vi "Analog_Hysteresis.vi"() -> ()   [LabVIEW 2011]
uses:
  <vilib>/Platform/TimedLoop/XDataNode/timing_clust.ctl
  <vilib>/Platform/TimedLoop/XDataNode/nitl_modes.ctl
  <vilib>/Platform/TimedLoop/XDataNode/wakeup.ctl
  <vilib>/Utility/error.llb/DialogType.ctl
  <vilib>/DAQmx/read.llb/DAQmx Read (Analog 2D DBL NChan NSamp).vi
  <vilib>/DAQmx/write.llb/DAQmx Write (Analog 1D DBL NChan 1Samp).vi
  <vilib>/DAQmx/create/channels.llb/DAQmx Create Channel (AI-Voltage-Basic).vi
  <vilib>/DAQmx/configure/timing.llb/DAQmx Timing (Sample Clock).vi
  <vilib>/Utility/file.llb/Write To Spreadsheet File (DBL).vi
  <vilib>/DAQmx/miscellaneous.llb/DAQmx Fill In Error Info.vi
  <vilib>/Platform/TimedLoop/XDataNode/XDataNode.xnode
  <vilib>/Platform/TimedLoop/XDataNode/XDNodeRunTimeDep.lvlib
panel:
  in  "Increase":bool
  in  "Decrease":bool
  out "Displacement input":T1(graph)
  out "XY Graph":cluster{"Y":dbl[], "Y":dbl[]}[](graph)
  in  "En H Inv":bool
  out "Time":dbl
  in  "Frequency 3":dbl=1.0
  in  "Amplitude":dbl[](array[numeric])=[0.0, 0.0, 0.0]
  out "Piezo driver input":T1(graph)
  out "Capacitive Sensor":T2(graph)
  in  "stop":bool
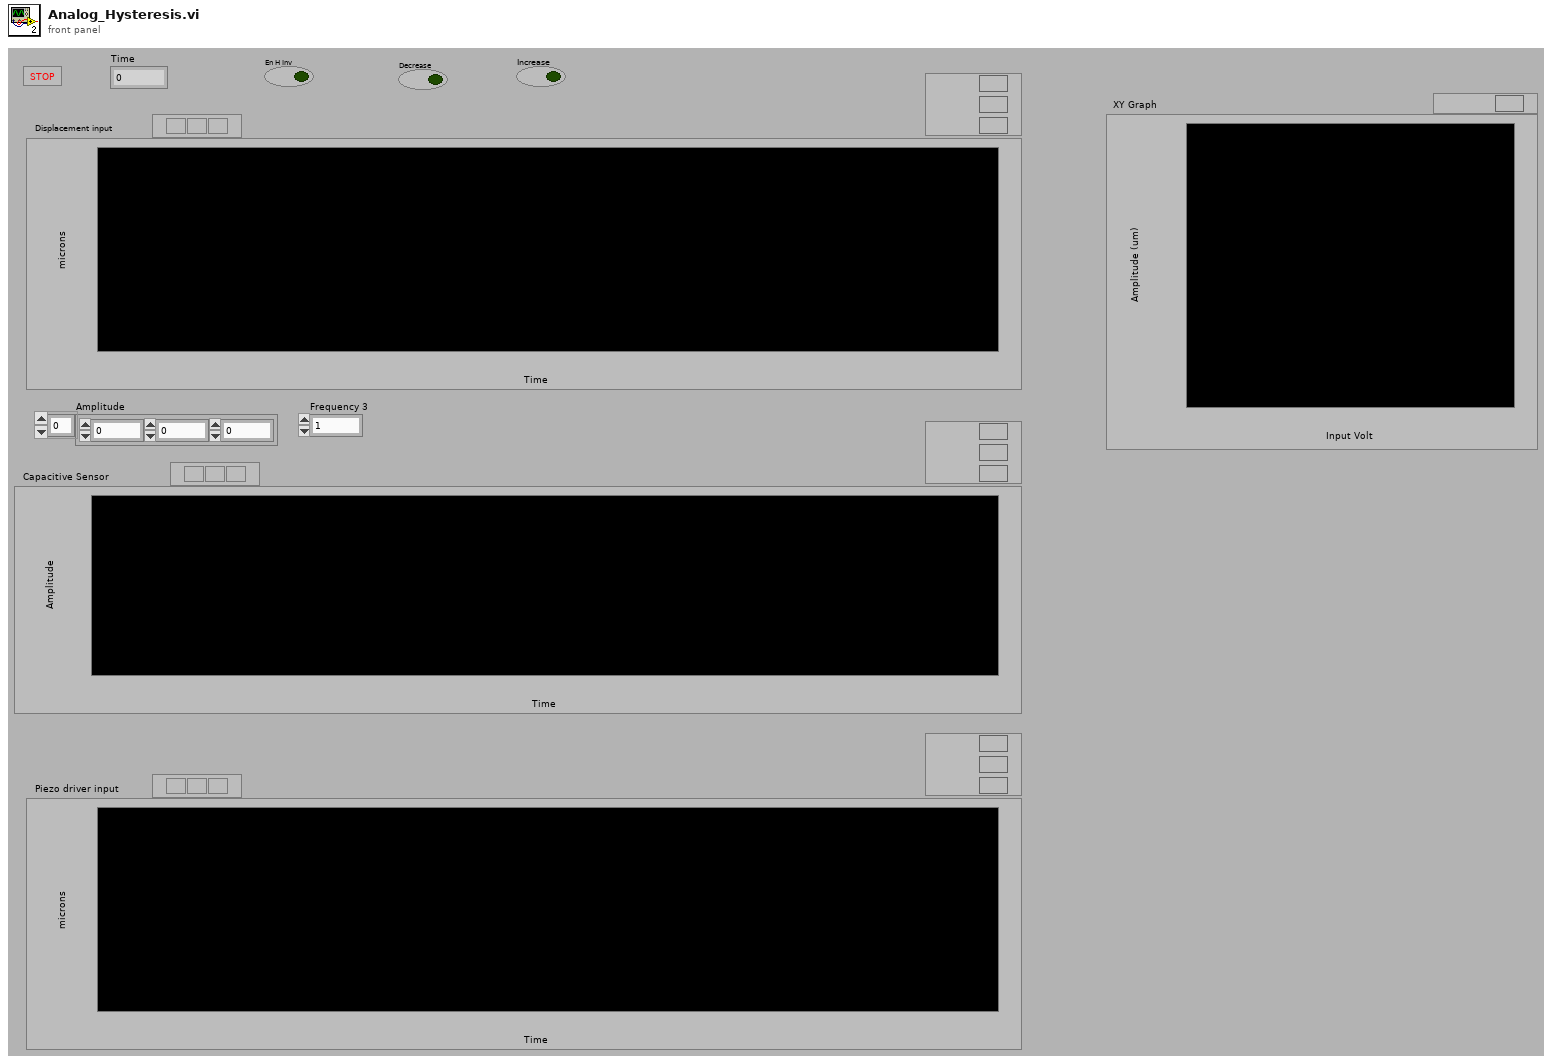
[diagram p1: front panel]
types:
  T1 = cluster{"dataOut[0]":dbl, "dataOut[1]":dbl, "dataOut[2]":dbl, "dataOut[3]":dbl, "dataOut[4]":dbl, "dataOut[5]":dbl, "dataOut[6]":dbl, "dataOut[7]":dbl, "dataOut[8]":dbl}
  T2 = cluster{"[0]":dbl, "[1]":dbl, "[2]":dbl, "[3]":dbl, "[4]":dbl, "[5]":dbl, "[6]":dbl, "[7]":dbl, "[8]":dbl}
  T3 = typedef "DialogType.ctl" = u16
  T4 = cluster{dbl[][], dbl[][], dbl[][], dbl[][], dbl, dbl, dbl}
  T5 = typedef "XDNodeRunTimeDep.lvlib/timing_clust.ctl" = cluster{"Expected End [f-1]":u64, "Actual End [f-1]":u64, "Finished Late? [f-1]":bool, "Expected End [i-1]":u64, "Actual End [i-1]":u64, "Finished Late? [i-1]":bool, "Expected Start [i]":u64, "Actual Start [i]":u64, "Expected Start [f]":u64, "Actual Start [f]":u64, "Source Name":string, "Structure Name":string, "Period":i64, "Deadline":i64, "Offset":i64, "Start":i64, "Priority":i32, "Timeout":i32, "Mode":T6, "Wakeup Reason":T7, "Error":errorcluster, "Source Type":string, "Secondary Source Type":string, "Global End Time":u64, "Global Start Time":u64, "Frame Duration":u64, "Iteration Duration":u64, "Assigned CPU":i32, "I/O Scan Engine Mode":u32}
  T6 = typedef "XDNodeRunTimeDep.lvlib/nitl_modes.ctl" = enum32{"No Change", "Process missed periods, maintain original phase", "Discard missed periods, maintain original phase", "Process missed periods, ignore original phase", "Discard missed periods, ignore original phase"}
  T7 = typedef "XDNodeRunTimeDep.lvlib/wakeup.ctl" = enum32{"Normal", "Aborted", "Asynchronous wakeup", "Timing source error", "Timed loop error", "Timeout"}
  T8 = cluster{"xyz[0]":dbl, "xyz[1]":dbl, "xyz[2]":dbl, "xyz[3]":dbl, "xyz[4]":dbl, "xyz[5]":dbl, "xyz[6]":dbl, "xyz[7]":dbl, "xyz[8]":dbl}
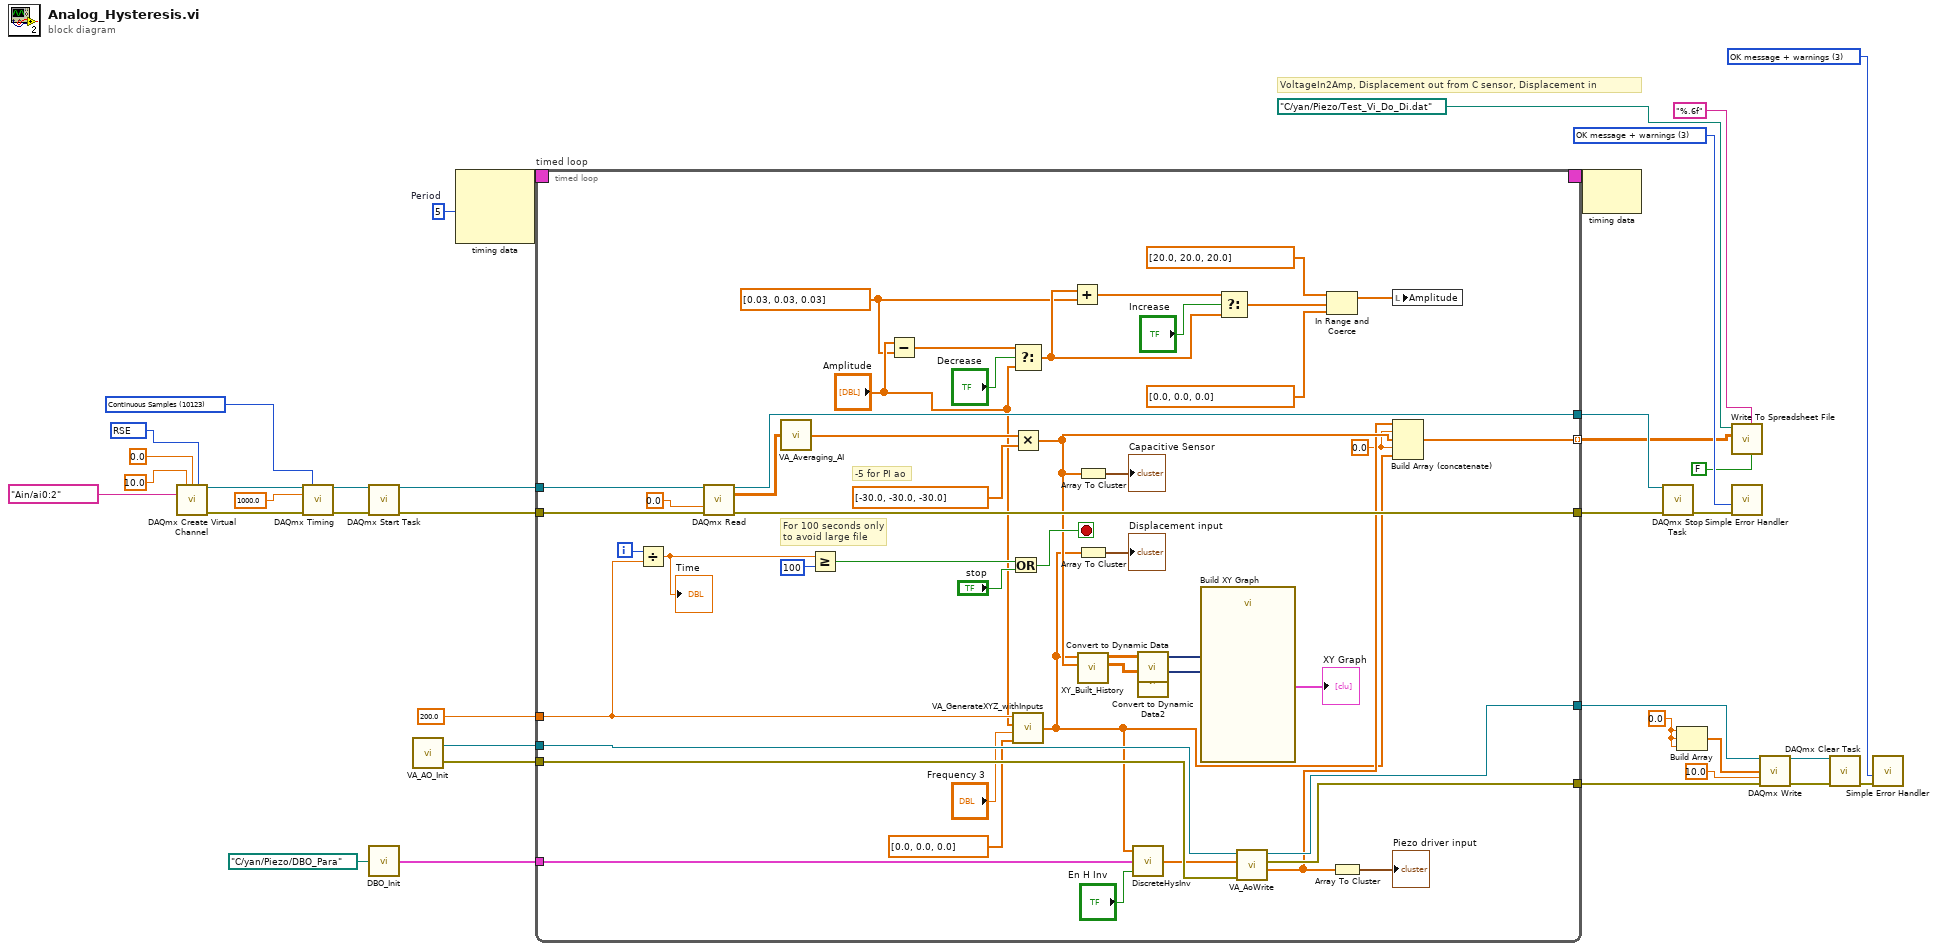
[diagram p0: block diagram]
diagram:
  w12 = 0.0 ("element")
  w15 = T3 3 items=["no dialog", "OK message", "continue or stop message", "OK message + warnings", "continue/stop + warnings"] ("type of dialog (OK msg:1)")
  w22 = T3 3 items=["no dialog", "OK message", "continue or stop message", "OK message + warnings", "continue/stop + warnings"] ("type of dialog (OK msg:1)")
  w29 = 10123 items=["Finite Samples"=10178, "Continuous Samples"=10123, "Hardware Timed Single Point"=12522] ("sample mode")
  w34 = 10083 items=["default"=-1, "RSE"=10083, "NRSE"=10078, "Differential"=10106, "Pseudodifferential"=12529] ("input terminal configuration")
  w35 = i64 5  # Period
  # "VoltageIn2Amp, Displacement out from C sensor, Displacement in"
  n1 = call-poly <vilib>:"DAQmx Create Virtual Channel.vi"("maximum value"=10.0, "minimum value"=0.0, "input terminal configuration"=w34, "physical channels"=tag "Ain/ai0:2") -> ("task out"=w31:refnum<k21>, "error out"=w30:errorcluster)  [unwired: 10 in]
  n2 = call-poly <vilib>:"DAQmx Timing.vi"("task/channels in"=w31, "sample mode"=w29, "rate"=1000.0, "error in"=w30) -> ("task out"=w27:refnum<k21>, "error out"=w26:errorcluster)  [unwired: 10 in]
  n3 = call <vilib>:"DAQmx Start Task.vi"("task/channels in"=w27, "error in"=w26) -> ("task out"=w24:refnum<k21>, "error out"=w23:errorcluster)  [unwired: 12 in]
  n4 = call "DBO_Init.vi"("base path"=path "C:/yan/Piezo/DBO_Para") -> ("DBO_Para"=w1:T4)
  n5 = call "VA_AO_Init.vi"() -> ("error out"=w8:errorcluster, "task out"=w9:refnum<k21>)
  n6 = node-c288(w35) -> (w37:T5)  [unwired: 2 out]
  n7 = timed-loop "timed loop" {
    timing: w37 -> [_]
    timing-out: [_] -> w36
    tunnel: w24 -> [w81]
    tunnel: w23 -> [w80]
    tunnel: [w79] -> w20
    tunnel: [w78] -> w19
    tunnel: [w74] -> w11
    tunnel: [w73] -> w10
    tunnel: w9 -> [w76]
    tunnel: w8 -> [w75]
    tunnel: 200.0 ("SampleFrequency") -> [w64]
    tunnel: [w68] -> w3 mode=indexing
    tunnel: w1 -> [w38]
    i -> [w65]
    stop <- w63 stop-if-true
    w39 = dbl[] [0.03, 0.03, 0.03] ("y")
    w51 = 0.0 ("timeout")
    # "For 100 seconds only\nto avoid large file"
    # "-5 for PI ao"
    n8 = Divide(x=w65, y=w64) -> (x/y=w66:dbl)
    "Time" <- w66
    n9 = call-poly <vilib>:"DAQmx Read.vi"("task/channels in"=w81, "timeout"=0.0, "error in"=w80) -> ("task out"=w78:refnum<k21>, "data"=w70:dbl[][], "error out"=w79:errorcluster)  [unwired: 10 in]
    n10 = call "VA_Averaging_AI.vi"("AnalogIn"=w70) -> ("Anolog XYZ"=w69:dbl[])
    n11 = Greater Or Equal?(x=w66, y=100) -> (x >= y?=w62:bool)
    n12 = Subtract(x="Amplitude", y=w39) -> (x-y=w48:dbl[])
    n13 = Or(x=w62, y="stop") -> (x .or. y?=w63:bool)
    n14 = Select(t=w48, s="Decrease", f="Amplitude") -> (s? t:f=w44:dbl[])
    n15 = Multiply(x=w69, y=dbl[] [-30.0, -30.0, -30.0]) -> (x*y=w54:dbl[])
    n16 = call "VA_GenerateXYZ_withInputs.vi"("Bias"=dbl[] [0.0, 0.0, 0.0] ("Amplitude"), "Frequency"="Frequency 3", "Amplitude"="Amplitude", "SampleFrequency"=w64) -> ("xyz"=w50:dbl[])
    n17 = Add(x=w44, y=w39) -> (x+y=w46:dbl[])
    n18 = Array To Cluster(array=w54) -> (cluster=→"Capacitive Sensor":T2)
    n19 = Array To Cluster(array=w50) -> (cluster=→"Displacement input":T8)
    n20 = call "XY_Built_History.vi"("input x"=w50, "input y"=w54) -> ("xo"=w58:sgl[][], "yo"=w56:sgl[][])  [unwired: 6 in]
    n21 = call "DiscreteHysInv.vi"("En H Inv"="En H Inv", "DBO Para"=w38, "input Yi"=w50) -> ("Xi"=w61:dbl[])
    n22 = call "Convert to Dynamic Data"("2D Array"=w58) -> ("Dynamic Data Type"=w57:dynamicdata)  [unwired: 3 in]
    n23 = call "Convert to Dynamic Data2"("2D Array"=w56) -> ("Dynamic Data Type"=w55:dynamicdata)  [unwired: 3 in]
    n24 = call "Build XY Graph"("Y Input"=w55, "X Input"=w57) -> ("XY Graph"=→"XY Graph":cluster{"Y":dbl[], "Y":dbl[]}[])  [unwired: 3 in, 6 out]
    n25 = Select(t=w46, s="Increase", f=w44) -> (s? t:f=w43:dbl[])
    n26 = call "VA_AoWrite.vi"("error in"=w75, "data"=w61, "task/channels in"=w76) -> ("dataOut"=w53:dbl[], "error out"=w73:errorcluster, "task out"=w74:refnum<k21>)  [unwired: 2 in]
    n27 = In Range and Coerce(upper limit=dbl[] [20.0, 20.0, 20.0], x=w43, lower limit=dbl[] [0.0, 0.0, 0.0] ("upper limit")) -> (coerced(x)=w40:dbl[])  [unwired: 1 out]
    n28 = Array To Cluster(array=w53) -> (cluster=→"Piezo driver input":T1)
    n29 = local write "Amplitude"(w40) -> ()
    n30 = Build Array (concatenate)(w53, w51, w54, w51, w50) -> (w68:dbl[])
  }
  n31 = node-c288(w36) -> ()  [unwired: 1 out]
  n32 = call <vilib>:"DAQmx Stop Task.vi"("task/channels in"=w19, "error in"=w20) -> ("error out"=w21:errorcluster)  [unwired: 12 in, 1 out]
  n33 = Build Array(w12, w12, w12) -> (w13:dbl[])
  n34 = call-poly <vilib>:"Write To Spreadsheet File.vi"("transpose? (no:F)"=FALSE, "format (%.3f)"="%.6f" ("format (%d)"), "2D data"=w3, "file path (dialog if empty)"=path "C:/yan/Piezo/Test_Vi_Do_Di.dat") -> ()  [unwired: 4 in, 1 out]
  n35 = call <vilib>:"Simple Error Handler.vi"("type of dialog (OK msg:1)"=w22, "error in (no error)"=w21) -> ()  [unwired: 3 in, 5 out]
  n36 = call-poly <vilib>:"DAQmx Write.vi"("task/channels in"=w11, "data"=w13, "timeout"=10.0, "error in"=w10) -> ("task out"=w17:refnum<k21>, "error out"=w16:errorcluster)  [unwired: 9 in, 1 out]
  n37 = call <vilib>:"DAQmx Clear Task.vi"("task in"=w17, "error in"=w16) -> ("error out"=w14:errorcluster)  [unwired: 13 in]
  n38 = call <vilib>:"Simple Error Handler.vi"("type of dialog (OK msg:1)"=w15, "error in (no error)"=w14) -> ()  [unwired: 3 in, 5 out]
